vi "OutputActuators.vi"   [LabVIEW 2020]
doc: "This VI sends commands to the arm subsystem."
uses:
  GlobalActuators.vi
  GRNF_CTREMotor.vi
types:
  T1 = enum16{"No Changed Output", "New Normal Output", "New Testing Output"}
  T2 = typedef "WPI_MotorControlDeviceRef.ctl" = cluster{"DeviceStatus":errorcluster, "Type":T3, "PWM":cluster{"PWM Channel":T4, "DeadBand":T5}, "CAN":cluster{"Device Number":u8, "SetOutput VI Ref":variant, "GetOutput VI Ref":variant, "Enable VI Ref":variant, "Disable VI Ref":variant, "Data":variant}, "Invert":bool, "DIO PWM":cluster{"PWM \"Enable\" Channel":T4, "DIOChannel":T6, "PWM Rate":dbl}}
  T3 = typedef "WPI_MotorControlType.ctl" = enum16{"PWM", "CAN", "DIO PWM"}
  T4 = typedef "FPGA_DIOPWMChannel.ctl" = enum8{"PWM 0", "PWM 1", "PWM 2", "PWM 3", "PWM 4", "PWM 5", "PWM 6", "PWM 7", "PWM 8", "PWM 9", "PWM MXP 0", "PWM MXP 1", "PWM MXP 2", "PWM MXP 3", "PWM MXP 4", "PWM MXP 5", "PWM MXP 6", "PWM MXP 7", "PWM MXP 8", "PWM MXP 9", "Invalid"}
  T5 = typedef "WPI_PWMDeadband.ctl" = cluster{"Name":string, "maxPositivePwm":i32, "minPositivePwm":i32, "centerPwm":i32, "maxNegativePwm":i32, "minNegativePwm":i32, "angularRange":u16}
  T6 = typedef "FPGA_DIOChannel.ctl" = enum8{"DIO 0", "DIO 1", "DIO 2", "DIO 3", "DIO 4", "DIO 5", "DIO 6", "DIO 7", "DIO 8", "DIO 9", "DIO MXP 0", "DIO MXP 1", "DIO MXP 2", "DIO MXP 3", "DIO MXP 4", "DIO MXP 5", "DIO MXP 6", "DIO MXP 7", "DIO MXP 8", "DIO MXP 9", "DIO MXP 10", "DIO MXP 11", "DIO MXP 12", "DIO MXP 13", "DIO MXP 14", "DIO MXP 15", "SPI Port CS1", "SPI Port CS2", "SPI Port CS3", "SPI Port MISO", "SPI Port MOSI", "Invalid"}
  T7 = typedef "WPI_SolenoidDevRef.ctl" = cluster{"DevStatus":errorcluster, "Pneumatics Control Module":u8, "Forward Solenoid Channel":T8, "Reverse Solenoid Channel":T8}
  T8 = typedef "WPI_SolenoidChannel.ctl" = enum8{"Solenoid 0", "Solenoid 1", "Solenoid 2", "Solenoid 3", "Solenoid 4", "Solenoid 5", "Solenoid 6", "Solenoid 7", "Solenoid 8", "Solenoid 9", "Solenoid 10", "Solenoid 11", "Solenoid 12", "Solenoid 13", "Solenoid 14", "Solenoid 15", "Invalid"}
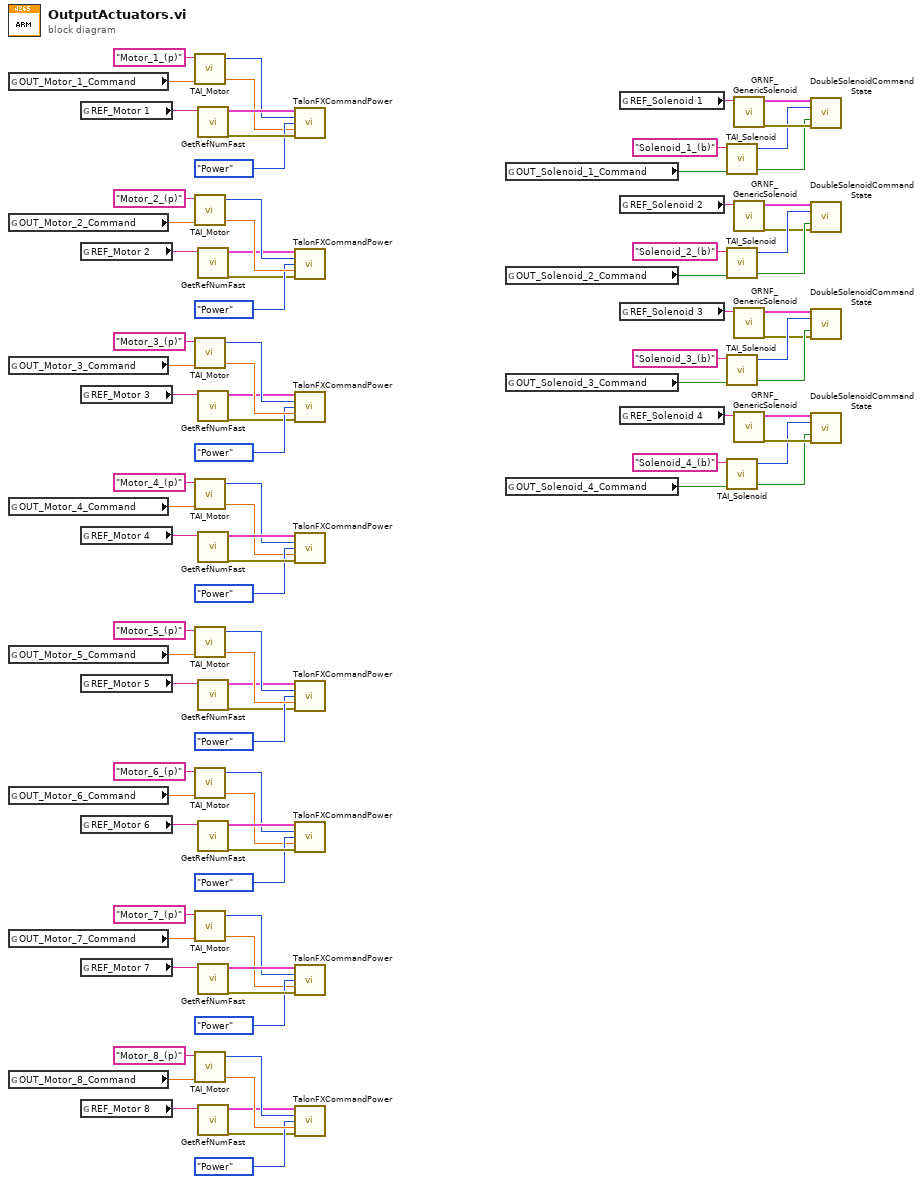
[diagram p0: block diagram]
diagram:
  n1 = global read "GlobalActuators.vi" "OUT_Motor_1_Command"() -> (w92:dbl)
  n2 = global read "GlobalActuators.vi" "OUT_Motor_2_Command"() -> (w77:dbl)
  n3 = global read "GlobalActuators.vi" "OUT_Motor_3_Command"() -> (w61:dbl)
  n4 = global read "GlobalActuators.vi" "OUT_Motor_4_Command"() -> (w76:dbl)
  n5 = global read "GlobalActuators.vi" "OUT_Motor_5_Command"() -> (w29:dbl)
  n6 = global read "GlobalActuators.vi" "OUT_Motor_6_Command"() -> (w44:dbl)
  n7 = global read "GlobalActuators.vi" "OUT_Motor_7_Command"() -> (w60:dbl)
  n8 = global read "GlobalActuators.vi" "OUT_Motor_8_Command"() -> (w45:dbl)
  n9 = global read "GlobalActuators.vi" "REF_Motor 1"() -> (w90:string)
  n10 = global read "GlobalActuators.vi" "REF_Motor 2"() -> (w79:string)
  n11 = global read "GlobalActuators.vi" "REF_Motor 3"() -> (w63:string)
  n12 = global read "GlobalActuators.vi" "REF_Motor 4"() -> (w74:string)
  n13 = global read "GlobalActuators.vi" "REF_Motor 5"() -> (w31:string)
  n14 = global read "GlobalActuators.vi" "REF_Motor 6"() -> (w42:string)
  n15 = global read "GlobalActuators.vi" "REF_Motor 7"() -> (w58:string)
  n16 = global read "GlobalActuators.vi" "REF_Motor 8"() -> (w47:string)
  n17 = call "TAI_Motor.vi"("Normal Output"=w92, "Actuator Name"="Motor_1_(p)") -> ("Interlocked Output"=w85:dbl, "Testing Mode"=w86:T1)  [unwired: 3 in]
  n18 = call "TAI_Motor.vi"("Normal Output"=w77, "Actuator Name"="Motor_2_(p)") -> ("Interlocked Output"=w84:dbl, "Testing Mode"=w83:T1)  [unwired: 3 in]
  n19 = call "TAI_Motor.vi"("Normal Output"=w61, "Actuator Name"="Motor_3_(p)") -> ("Interlocked Output"=w68:dbl, "Testing Mode"=w67:T1)  [unwired: 3 in]
  n20 = call "TAI_Motor.vi"("Normal Output"=w76, "Actuator Name"="Motor_4_(p)") -> ("Interlocked Output"=w69:dbl, "Testing Mode"=w70:T1)  [unwired: 3 in]
  n21 = call "TAI_Motor.vi"("Normal Output"=w29, "Actuator Name"="Motor_5_(p)") -> ("Interlocked Output"=w36:dbl, "Testing Mode"=w35:T1)  [unwired: 3 in]
  n22 = call "TAI_Motor.vi"("Normal Output"=w44, "Actuator Name"="Motor_6_(p)") -> ("Interlocked Output"=w37:dbl, "Testing Mode"=w38:T1)  [unwired: 3 in]
  n23 = call "TAI_Motor.vi"("Normal Output"=w60, "Actuator Name"="Motor_7_(p)") -> ("Interlocked Output"=w53:dbl, "Testing Mode"=w54:T1)  [unwired: 3 in]
  n24 = call "TAI_Motor.vi"("Normal Output"=w45, "Actuator Name"="Motor_8_(p)") -> ("Interlocked Output"=w52:dbl, "Testing Mode"=w51:T1)  [unwired: 3 in]
  n25 = call-poly "GetRefNumFast.vi"("RefNum Name"=w90) -> ("Error"=w88:errorcluster, "Device Reference"=w89:T2)  [unwired: 5 in]
  n26 = call-poly "GetRefNumFast.vi"("RefNum Name"=w79) -> ("Error"=w81:errorcluster, "Device Reference"=w80:T2)  [unwired: 5 in]
  n27 = call-poly "GetRefNumFast.vi"("RefNum Name"=w63) -> ("Error"=w65:errorcluster, "Device Reference"=w64:T2)  [unwired: 5 in]
  n28 = call-poly "GetRefNumFast.vi"("RefNum Name"=w74) -> ("Error"=w72:errorcluster, "Device Reference"=w73:T2)  [unwired: 5 in]
  n29 = call-poly "GetRefNumFast.vi"("RefNum Name"=w31) -> ("Error"=w33:errorcluster, "Device Reference"=w32:T2)  [unwired: 5 in]
  n30 = call-poly "GetRefNumFast.vi"("RefNum Name"=w42) -> ("Error"=w40:errorcluster, "Device Reference"=w41:T2)  [unwired: 5 in]
  n31 = call-poly "GetRefNumFast.vi"("RefNum Name"=w58) -> ("Error"=w56:errorcluster, "Device Reference"=w57:T2)  [unwired: 5 in]
  n32 = call-poly "GetRefNumFast.vi"("RefNum Name"=w47) -> ("Error"=w49:errorcluster, "Device Reference"=w48:T2)  [unwired: 5 in]
  n33 = call "TalonFXCommandPower.vi"("Device Reference (in)"=w89, "Output Mode"=w86, "Control Mode"=enum16{"Safety", "Power"}."Power", "Power or Testing Power"=w85, "Error (in)"=w88) -> ()  [unwired: 11 in]
  n34 = call "TalonFXCommandPower.vi"("Device Reference (in)"=w80, "Output Mode"=w83, "Control Mode"=enum16{"Safety", "Power"}."Power", "Power or Testing Power"=w84, "Error (in)"=w81) -> ()  [unwired: 11 in]
  n35 = call "TalonFXCommandPower.vi"("Device Reference (in)"=w64, "Output Mode"=w67, "Control Mode"=enum16{"Safety", "Power"}."Power", "Power or Testing Power"=w68, "Error (in)"=w65) -> ()  [unwired: 11 in]
  n36 = call "TalonFXCommandPower.vi"("Device Reference (in)"=w73, "Output Mode"=w70, "Control Mode"=enum16{"Safety", "Power"}."Power", "Power or Testing Power"=w69, "Error (in)"=w72) -> ()  [unwired: 11 in]
  n37 = call "TalonFXCommandPower.vi"("Device Reference (in)"=w32, "Output Mode"=w35, "Control Mode"=enum16{"Safety", "Power"}."Power", "Power or Testing Power"=w36, "Error (in)"=w33) -> ()  [unwired: 11 in]
  n38 = call "TalonFXCommandPower.vi"("Device Reference (in)"=w41, "Output Mode"=w38, "Control Mode"=enum16{"Safety", "Power"}."Power", "Power or Testing Power"=w37, "Error (in)"=w40) -> ()  [unwired: 11 in]
  n39 = call "TalonFXCommandPower.vi"("Device Reference (in)"=w57, "Output Mode"=w54, "Control Mode"=enum16{"Safety", "Power"}."Power", "Power or Testing Power"=w53, "Error (in)"=w56) -> ()  [unwired: 11 in]
  n40 = call "TalonFXCommandPower.vi"("Device Reference (in)"=w48, "Output Mode"=w51, "Control Mode"=enum16{"Safety", "Power"}."Power", "Power or Testing Power"=w52, "Error (in)"=w49) -> ()  [unwired: 11 in]
  n41 = global read "GlobalActuators.vi" "OUT_Solenoid_1_Command"() -> (w28:bool)
  n42 = global read "GlobalActuators.vi" "OUT_Solenoid_2_Command"() -> (w15:bool)
  n43 = global read "GlobalActuators.vi" "OUT_Solenoid_3_Command"() -> (w1:bool)
  n44 = global read "GlobalActuators.vi" "OUT_Solenoid_4_Command"() -> (w14:bool)
  n45 = global read "GlobalActuators.vi" "REF_Solenoid 1"() -> (w26:string)
  n46 = global read "GlobalActuators.vi" "REF_Solenoid 2"() -> (w17:string)
  n47 = global read "GlobalActuators.vi" "REF_Solenoid 3"() -> (w3:string)
  n48 = global read "GlobalActuators.vi" "REF_Solenoid 4"() -> (w12:string)
  n49 = call "TAI_Solenoid.vi"("Normal Output"=w28, "Actuator Name"="Solenoid_1_(b)") -> ("Interlocked Output"=w22:bool, "Output Mode"=w23:T1)  [unwired: 3 in]
  n50 = call "TAI_Solenoid.vi"("Normal Output"=w15, "Actuator Name"="Solenoid_2_(b)") -> ("Interlocked Output"=w21:bool, "Output Mode"=w20:T1)  [unwired: 3 in]
  n51 = call "TAI_Solenoid.vi"("Normal Output"=w1, "Actuator Name"="Solenoid_3_(b)") -> ("Interlocked Output"=w7:bool, "Output Mode"=w6:T1)  [unwired: 3 in]
  n52 = call "TAI_Solenoid.vi"("Normal Output"=w14, "Actuator Name"="Solenoid_4_(b)") -> ("Interlocked Output"=w8:bool, "Output Mode"=w9:T1)  [unwired: 3 in]
  n53 = call "GRNF_GenericSolenoid.vi"("RefNum Name"=w26) -> ("Error"=w24:errorcluster, "Device Reference"=w25:T7)  [unwired: 5 in]
  n54 = call "GRNF_GenericSolenoid.vi"("RefNum Name"=w17) -> ("Error"=w19:errorcluster, "Device Reference"=w18:T7)  [unwired: 5 in]
  n55 = call "GRNF_GenericSolenoid.vi"("RefNum Name"=w3) -> ("Error"=w5:errorcluster, "Device Reference"=w4:T7)  [unwired: 5 in]
  n56 = call "GRNF_GenericSolenoid.vi"("RefNum Name"=w12) -> ("Error"=w10:errorcluster, "Device Reference"=w11:T7)  [unwired: 5 in]
  n57 = call "DoubleSolenoidCommandState.vi"("Device Reference (in)"=w25, "Output Mode"=w23, "State [True, False]"=w22, "Error (in)"=w24) -> ()  [unwired: 12 in]
  n58 = call "DoubleSolenoidCommandState.vi"("Device Reference (in)"=w18, "Output Mode"=w20, "State [True, False]"=w21, "Error (in)"=w19) -> ()  [unwired: 12 in]
  n59 = call "DoubleSolenoidCommandState.vi"("Device Reference (in)"=w4, "Output Mode"=w6, "State [True, False]"=w7, "Error (in)"=w5) -> ()  [unwired: 12 in]
  n60 = call "DoubleSolenoidCommandState.vi"("Device Reference (in)"=w11, "Output Mode"=w9, "State [True, False]"=w8, "Error (in)"=w10) -> ()  [unwired: 12 in]
